vi "Write_to_XML_File.vi"(11 "2D-Array":dbl[][](array[numeric])) -> ()   [LabVIEW 2011]
uses:
  <vilib>/Utility/xml.llb/Write to XML File(string).vi
panel:
  out "XML Output":string
  out "XML File Path":path
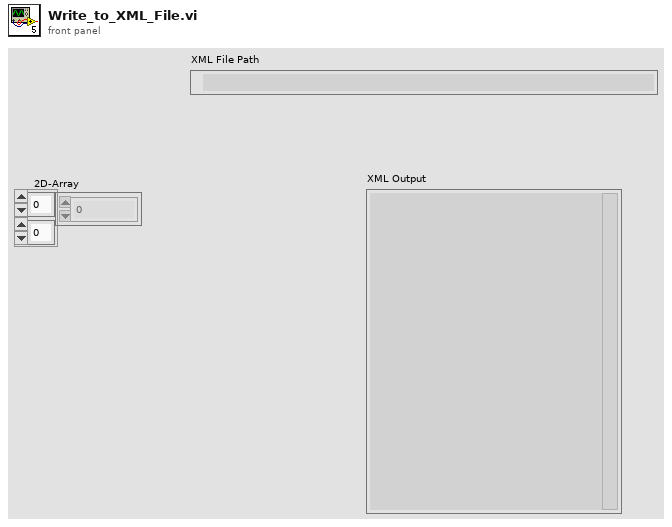
[diagram p1: front panel]
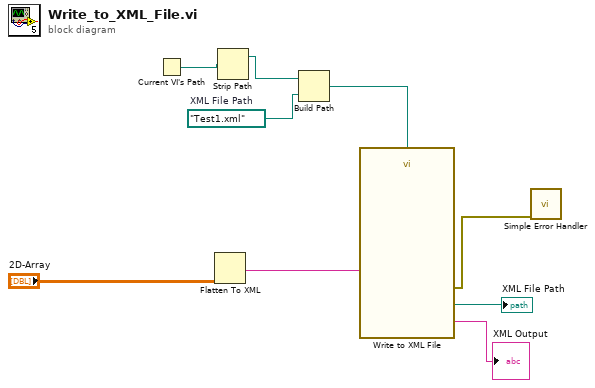
[diagram p0: block diagram]
diagram:
  w4 = path "Test1.xml"  # XML File Path
  n1 = Current VI's Path() -> (path=w2:path)
  n2 = Flatten To XML(anything="2D-Array") -> (xml string=w8:string)
  n3 = Strip Path(path=w2) -> (stripped path=w1:path)  [unwired: 1 out]
  n4 = Build Path(base path=w1, name or relative path=w4) -> (appended path=w9:path)
  n5 = call-poly <vilib>:"Write to XML File.vi"("XML Input"=w8, "XML File Path"=w9) -> ("error out"=w5:errorcluster, "XML String"=→"XML Output":string, "XML File Path(duplicate)"=→"XML File Path":path)  [unwired: 7 in]
  n6 = call <vilib>:"Simple Error Handler.vi"("error in (no error)"=w5) -> ()  [unwired: 4 in, 5 out]
